vi "Laplace CDF.vi"(9 "b":dbl=1.0, 10 "a":dbl=1.0, 11 "x":dbl) -> (0 "error":i32, 3 "cdf(x)":dbl=0.18393972058572117)   [LabVIEW 2018, in "NI_Gmath.lvlib"]
doc: "Computes the continuous cumulative distribution function (CDF), or the probability that the random variate X, where X describes the selected distribution type, has a value less than or equal to <B>x</B>. You must manually select the polymorphic instance to use."
uses:
  NI_Gmath.lvlib
  st_error_code.ctl
panel:
  # "Laplace CDF"
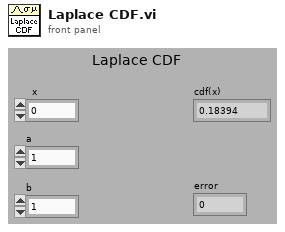
[diagram p1: front panel]
types:
  T1 = typedef "NI_Gmath.lvlib/st_error_code.ctl" = i32
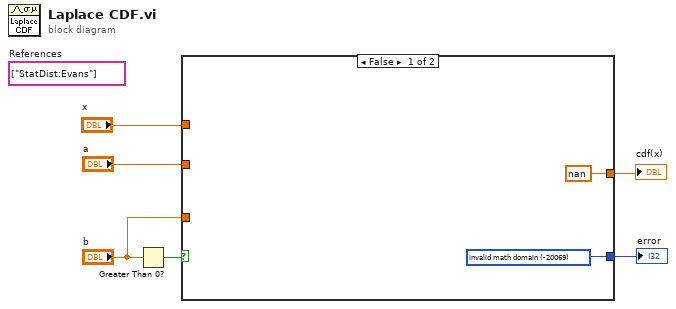
[diagram p0: block diagram]
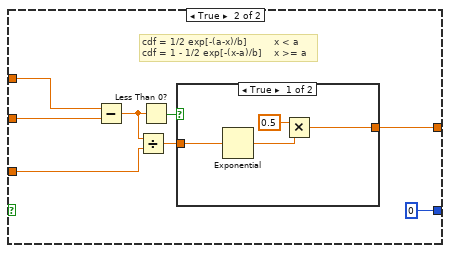
[diagram p2: hidden frame]
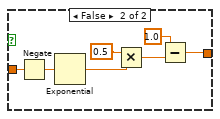
[diagram p3: hidden frame]
diagram:
  (unwired) string[] ["StatDist:Evans"]  # References
  n1 = Greater Than 0?(x="b") -> (x > 0?=w3:bool)
  n2 = case shown="False" w3 {
    tunnel: "b" -> [_ w13]
    tunnel: [w7 0 ("invalid math domain")] -> w1
    tunnel: [nan w11] -> w2
    tunnel: "x" -> [_ w15]
    tunnel: "a" -> [_ w14]
    frame False {
      w7 = T1 -20069 items=["invalid math domain"=-20069, "Fourier interpolation size m >= n"=-20070, "empty array"=-20003] ("stat interp error code")
    }
    frame True {
      # "cdf = 1/2 exp[-(a-x)/b]         x < a\ncdf = 1 - 1/2 exp[-(x-a)/b]    x >= a"
      n3 = Subtract(x=w15, y=w14) -> (x-y=w9:dbl)
      n4 = Divide(x=w9, y=w13) -> (x/y=w12:dbl)
      n5 = Less Than 0?(x=w9) -> (x < 0?=w10:bool)
      n6 = case shown="True" w10 {
        tunnel: w12 -> [w20 w27]
        tunnel: [w17 w22] -> w11
        frame True {
          n7 = Exponential(1:w20) -> (0:w19:dbl)
          n8 = Multiply(x=0.5, y=w19) -> (x*y=w17:dbl)
        }
        frame False {
          n9 = Negate(x=w27) -> (-x=w21:dbl)
          n10 = Exponential(1:w21) -> (0:w26:dbl)
          n11 = Multiply(x=0.5, y=w26) -> (x*y=w24:dbl)
          n12 = Subtract(x=1.0, y=w24) -> (x-y=w22:dbl)
        }
      }
    }
  }
  "cdf(x)" <- w2
  "error" <- w1
